vi "Get Physical Units.vi"() -> ()   [LabVIEW 2012, in "TD Tools.lvlib"]
uses:
  TD Tools.lvlib
  Custom Type/Physical Units.ctl
panel:
  out "错误输出":errorcluster
  in  "错误输入":errorcluster
  out "Physical Units":T1[](array[typedef])
  in  "Float or Array of Floats":variant
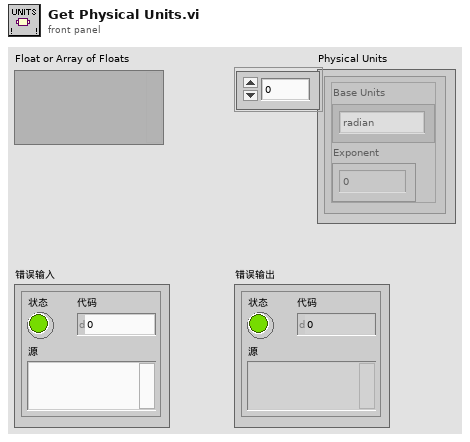
[diagram p1: front panel]
types:
  T1 = typedef "TD Tools.lvlib/Physical Units.ctl" = cluster{"Base Units":enum16{"radian", "steradian", "second", "meter", "kilogram", "ampere", "kelvin", "mole", "candela"}, "Exponent":dbl}
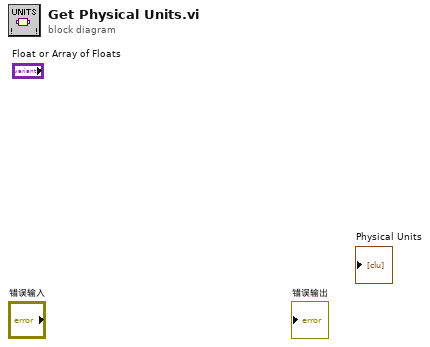
[diagram p0: block diagram]
diagram:
